vi "RESPONSE_LOGIC.vi"(11 "Array":string[][](array[string])) -> (3 "Not Found":i32[](array[numeric]))   [LabVIEW 2017]
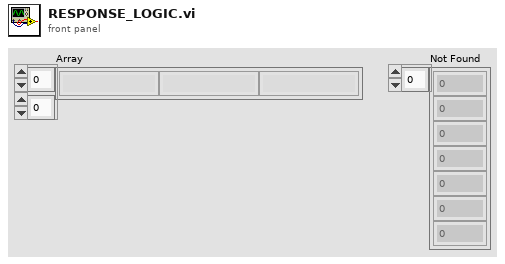
[diagram p1: front panel]
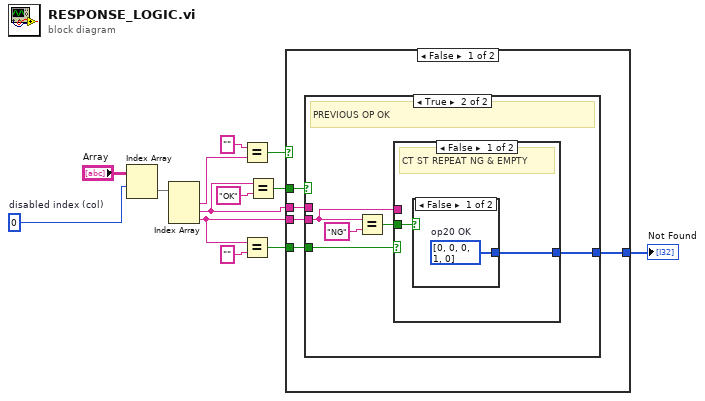
[diagram p0: block diagram]
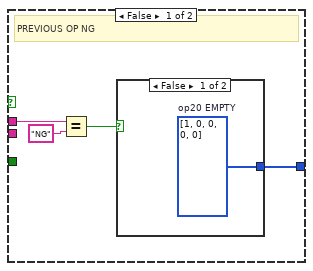
[diagram p2: hidden frame]
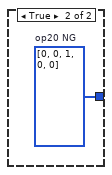
[diagram p3: hidden frame]
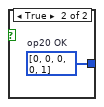
[diagram p4: hidden frame]
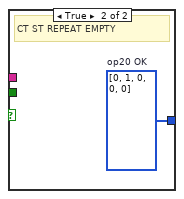
[diagram p5: hidden frame]
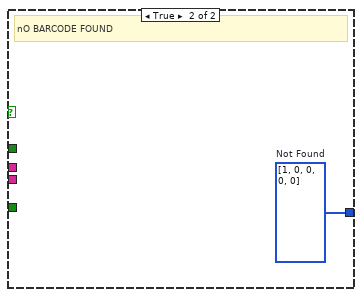
[diagram p6: hidden frame]
diagram:
  w3 = 0  # disabled index (col)
  n1 = Index Array(array="Array", index (row)=w3) -> (element=w2:string[])  [unwired: 1 in]
  n2 = Index Array(array=w2) -> (element #1=w13:string, element #2=w7:string, element #3=w5:string)  [unwired: 3 in]
  n3 = Equal?(x="", y=w13) -> (x = y?=w10:bool)
  n4 = Equal?(x=w5, y="") -> (x = y?=w6:bool)
  n5 = Equal?(x=w7, y="OK") -> (x = y?=w9:bool)
  n6 = case shown="False" w10 {
    tunnel: w9 -> [w18 _]
    tunnel: [w16 w35] -> w1
    tunnel: w7 -> [w17 _]
    tunnel: w6 -> [w15 _]
    tunnel: w5 -> [w14 _]
    frame False {
      n7 = case shown="True" w18 {
        tunnel: w17 -> [w22 _]
        tunnel: [w19 w25] -> w16
        tunnel: w15 -> [_ w29]
        tunnel: w14 -> [_ w27]
        frame False {
          # "PREVIOUS OP NG"
          n8 = Equal?(x=w22, y="NG") -> (x = y?=w20:bool)
          n9 = case shown="False" w20 {
            tunnel: [w23 w24] -> w19
            frame False {
              w23 = i32[] [1, 0, 0, 0, 0]  # op20 EMPTY
            }
            frame True {
              w24 = i32[] [0, 0, 1, 0, 0]  # op20 NG
            }
          }
        }
        frame True {
          # "PREVIOUS OP OK"
          n10 = Equal?(x=w27, y="NG") -> (x = y?=w26:bool)
          n11 = case shown="False" w29 {
            tunnel: w27 -> [_ _]
            tunnel: w26 -> [w31 _]
            tunnel: [w30 w34] -> w25
            frame False {
              # "CT ST REPEAT NG & EMPTY"
              n12 = case shown="False" w31 {
                tunnel: [w32 w33] -> w30
                frame False {
                  w32 = i32[] [0, 0, 0, 1, 0]  # op20 OK
                }
                frame True {
                  w33 = i32[] [0, 0, 0, 0, 1]  # op20 OK
                }
              }
            }
            frame True {
              w34 = i32[] [0, 1, 0, 0, 0]  # op20 OK
              # "CT ST REPEAT EMPTY"
            }
          }
        }
      }
    }
    frame True {
      w35 = i32[] [1, 0, 0, 0, 0]  # Not Found
      # "nO BARCODE FOUND"
    }
  }
  "Not Found" <- w1
